vi "createProjectItem.vi"(8 "error in (no error)":errorcluster, 10 "ProjectItemSelection":T1, 11 "IProjectItemFactory in":refnum<class "IProjectItemFactory.lvclass">) -> (0 "error out":errorcluster, 2 "ProjectItem":refnum<class "ProjectItem.lvclass">, 3 "IProjectItemFactory out":refnum<class "IProjectItemFactory.lvclass">)   [LabVIEW 2016, in "IProjectItemFactory.lvclass"]
uses:
  IProjectItemFactory.lvclass
  Typedefs/ProjectItemSelection.ctl
  ProjectItem/ProjectItem.lvclass
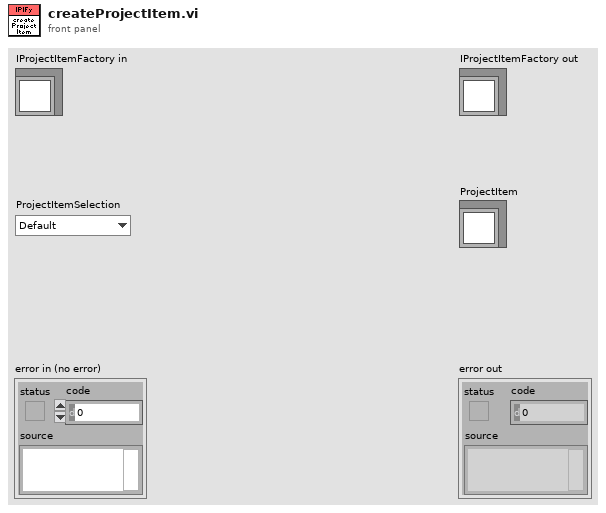
[diagram p1: front panel]
types:
  T1 = typedef "ProjectItemSelection.ctl" = enum16{"Default", "Dependencies", "Folder", "Library", "LVClass", "VI"}
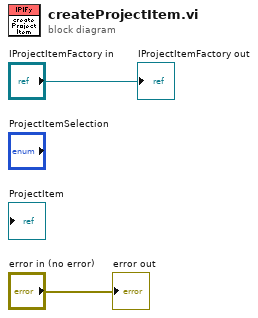
[diagram p0: block diagram]
diagram:
  "error out" <- "error in (no error)"
  "IProjectItemFactory out" <- "IProjectItemFactory in"
